vi "Bankomat.vi"() -> ()   [LabVIEW 2021]
uses:
  Stan.ctl
panel:
  in  "Enter":bool
  in  "PIN":string
  in  "Prawe przyciski":T1
  out "Prawe menu":T2
  in  "Lewe przyciski":T1
  out "Lewe menu":T2
  in  "Wprowadź karte":bool
  out "Ekran bankomatu":string
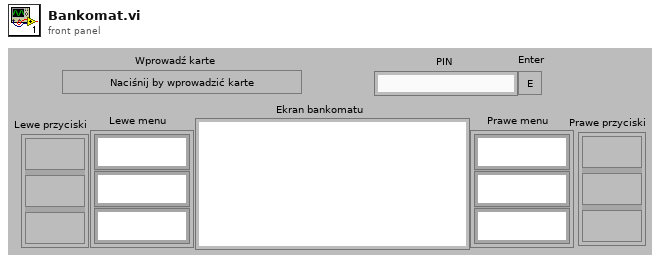
[diagram p1: front panel]
types:
  T1 = cluster{"Func Button":bool, "Func Button 2":bool, "Func Button 3":bool}
  T2 = cluster{"RFS String":string, "RFS String 2":string, "RFS String 3":string}
  T3 = typedef "Stan.ctl" = enum16{"Start", "Idle", "Deposit", "Withdraw", "FastCash", "None", "BalanceInquiry", "ReturnCard"}
  T4 = enum16{"CheckAccountNumber", "ReturnInfo", "Deposit", "Withdraw"}
  T5 = enum8{"Enabled", "Disabled", "Disabled and Grayed Out"}
  T6 = typedef "Konto.ctl" = cluster{"PIN":string, "Imie":string, "Nazwisko":string, "Balans":string}
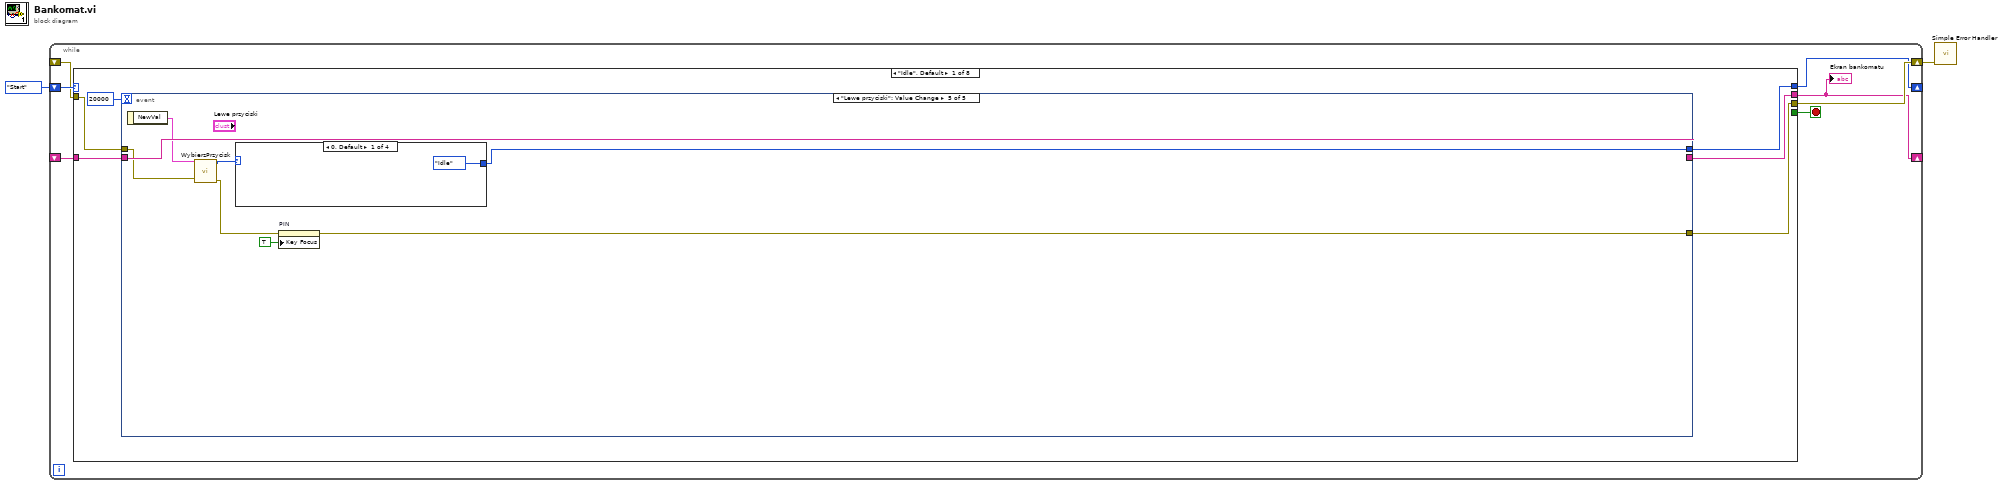
[diagram p0: block diagram]
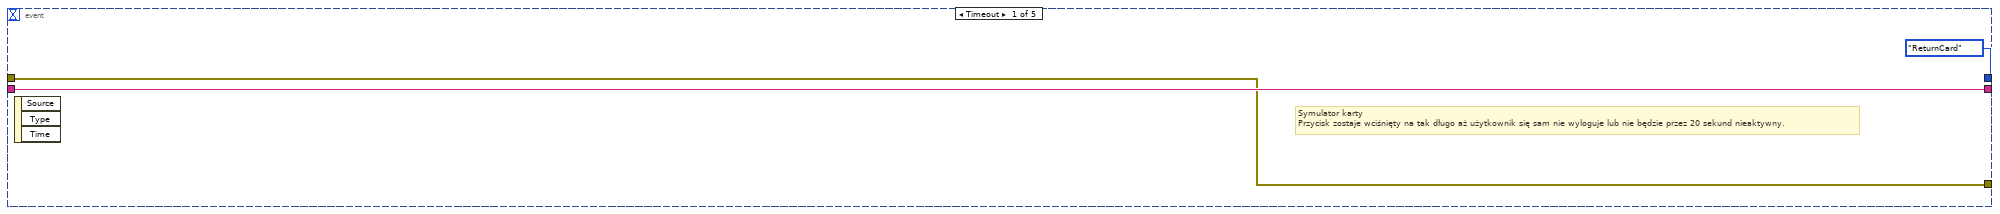
[diagram p2: hidden frame]
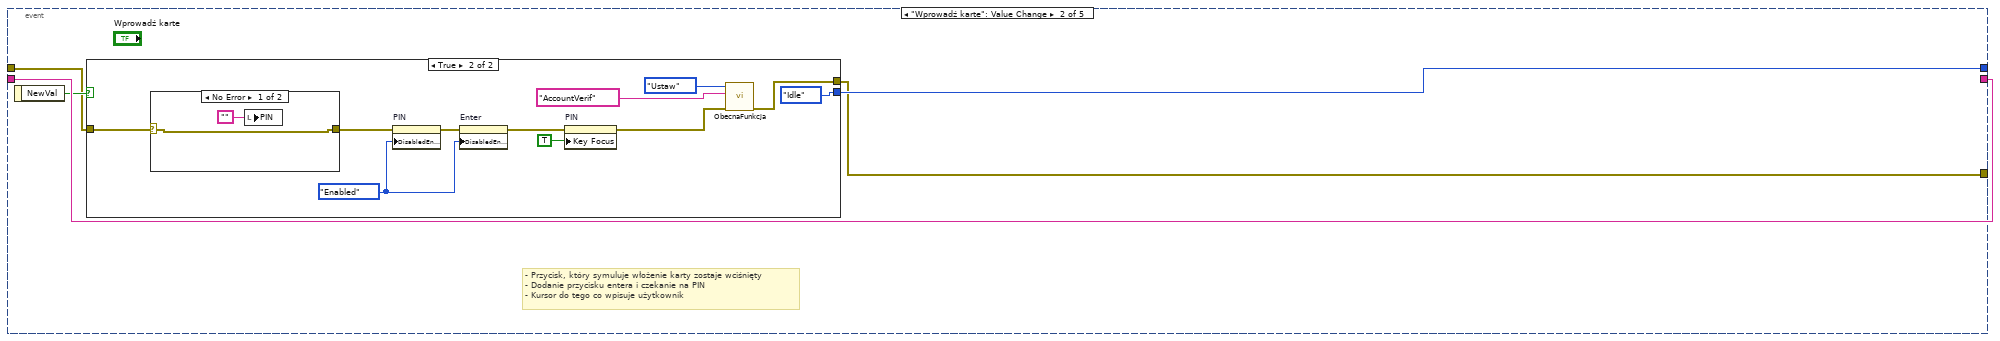
[diagram p3: hidden frame]
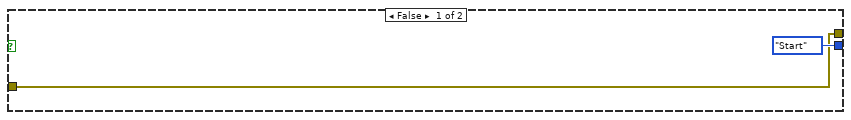
[diagram p4: hidden frame]
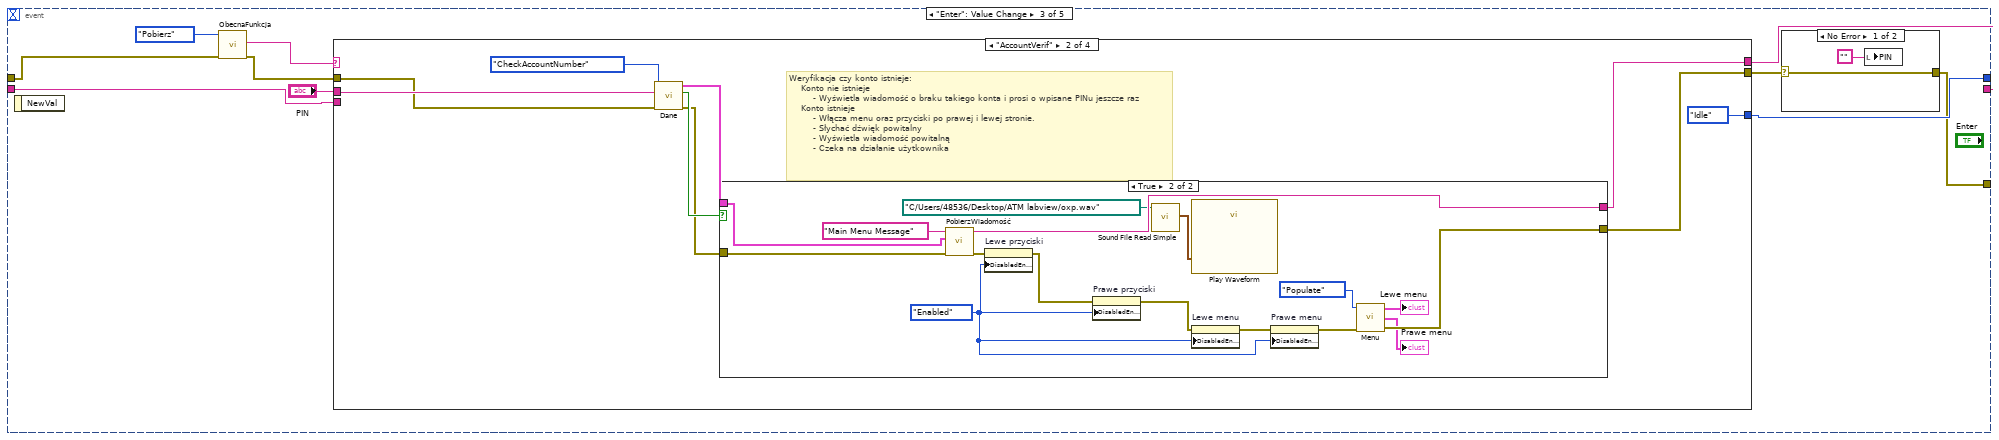
[diagram p6: hidden frame]
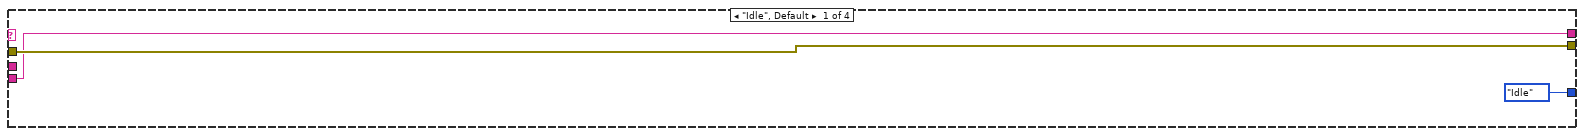
[diagram p8: hidden frame]
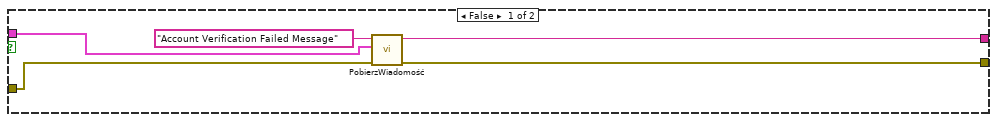
[diagram p9: hidden frame]
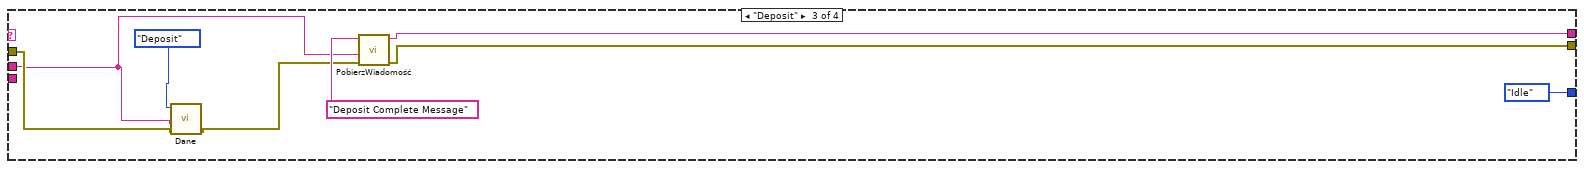
[diagram p10: hidden frame]
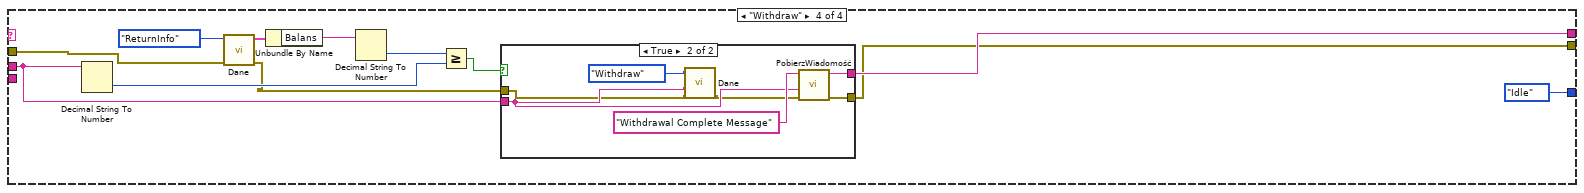
[diagram p11: hidden frame]
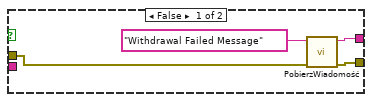
[diagram p12: hidden frame]
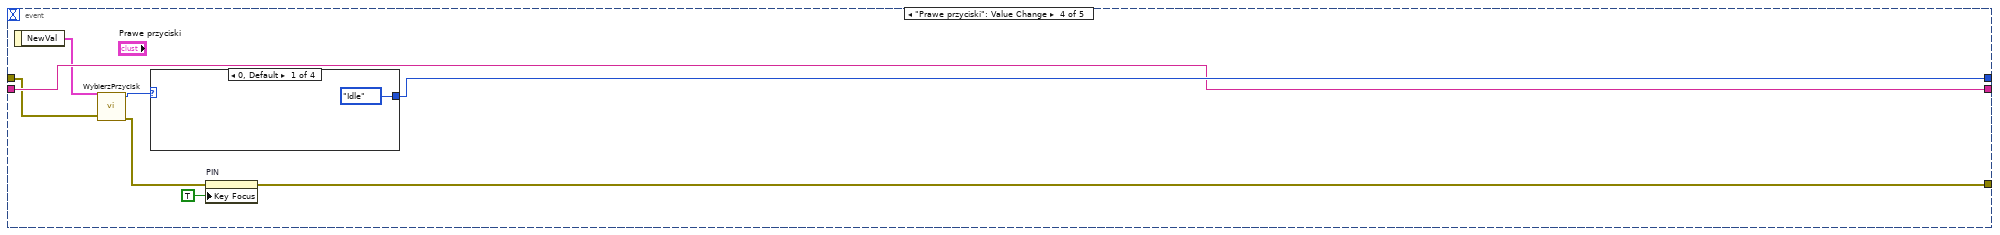
[diagram p13: hidden frame]
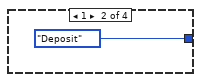
[diagram p14: hidden frame]
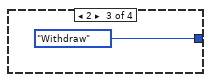
[diagram p15: hidden frame]
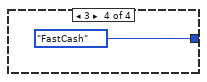
[diagram p16: hidden frame]
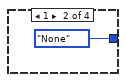
[diagram p17: hidden frame]
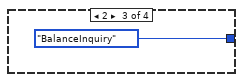
[diagram p18: hidden frame]
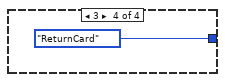
[diagram p19: hidden frame]
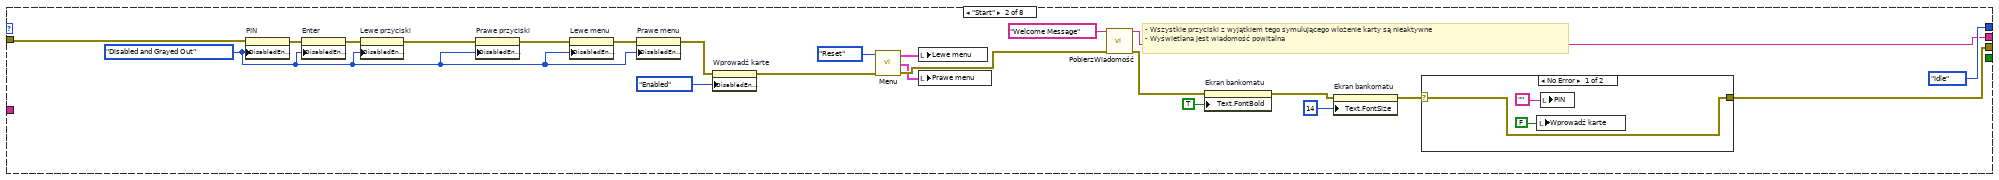
[diagram p20: hidden frame]
diagram:
  n1 = while {
    shift-right: [w3] -> _
    shift-left: Stan."Start" -> [w9]
    shift-right: [w8] -> w1
    shift-left: _ -> [w7]
    shift-right: [w5] -> _
    shift-left: _ -> [w4]
    stop <- w6 stop-if-true
    n2 = case shown="\"Idle\", Default" w9 {
      tunnel: [w12 Stan."Idle" _ Stan."Idle" Stan."Idle" Stan."Idle" Stan."Idle" Stan."Idle"] -> w3
      tunnel: [w13 w142 w180 w203 w212 w222 w241 w248] -> w8
      tunnel: w7 -> [w14 w141 w179 w202 w211 w219 w241 w247]
      tunnel: [_ _ TRUE _ _ _ _ _] -> w6
      tunnel: [w11 w153 w176 w204 w214 w223 "" ("Message") w249] -> w5
      tunnel: w4 -> [w10 _ _ _ _ _ _ _]
      frame "Idle", Default {
        n3 = event shown="[4] \"Lewe przyciski\": Value Change" {
          selector: _ -> [_ _ _ _ _]
          dyn-events: _ -> [_ _ _ _ _]
          timeout: 20000 -> [_ _ _ _ _]
          tunnel: [Stan."ReturnCard" w21 w49 w124 w136] -> w12
          tunnel: w14 -> [w16 w20 w44 w117 w129]
          tunnel: [w16 w19 w41 w121 w133] -> w13
          tunnel: [w17 w23 w46 w123 w135] -> w11
          tunnel: w10 -> [w17 w23 w45 w123 w135]
          event Timeout {
            # "Symulator karty \nPrzycisk zostaje wciśnięty na tak długo aż użytkownik się sam nie wyloguje lub nie będzie przez 20 sekund nieaktywny."
            n4 = event-data() -> ()  [unwired: 1 in, 3 out]
          }
          event "Wprowadź karte": Value Change {
            # "- Przycisk, który symuluje włożenie karty zostaje wciśnięty\n- Dodanie przycisku entera i czekanie na PIN \n- Kursor do tego co wpisuje użytkownik"
            n5 = event-data() -> ("NewVal"=w22:bool)  [unwired: 1 in]
            n6 = case shown="True" w22 {
              tunnel: [Stan."Start" Stan."Idle"] -> w21
              tunnel: w20 -> [w24 w29]
              tunnel: [w24 w27] -> w19
              frame False {
              }
              frame True {
                w36 = T5."Enabled" ("Disabled")
                n7 = case shown="No Error" w29 {
                  selector: w29 -> [w37 w39]
                  tunnel: [w37 w39] -> w28
                  frame No Error {
                    n8 = local write "PIN"("") -> ()
                  }
                  frame Error {
                  }
                }
                n9 = property on="PIN" class="Str"(error in=w28, "DisabledEnum"=w36) -> (error out=w32:errorcluster)  [unwired: 1 in, 1 out]
                n10 = property on="Enter" class="Bool"(error in=w32, "DisabledEnum"=w36) -> (error out=w31:errorcluster)  [unwired: 1 in, 1 out]
                n11 = property on="PIN" class="Str"(error in=w31, "Key Focus"=TRUE) -> (error out=w30:errorcluster)  [unwired: 1 in, 1 out]
                n12 = call "ObecnaFunkcja.vi"("error in"=w30, "Funkcja wejścia"="AccountVerif" ("Function In"), "Akcja"=enum16{"Ustaw", "Pobierz"}."Ustaw") -> ("error out"=w27:errorcluster)  [unwired: 7 in, 1 out]
              }
            }
          }
          event "Enter": Value Change {
            n13 = event-data() -> ()  [unwired: 1 in, 1 out]
            n14 = call "ObecnaFunkcja.vi"("error in"=w44, "Akcja"=enum16{"Ustaw", "Pobierz"}."Pobierz") -> ("error out"=w43:errorcluster, "Funkcja wyjścia"=w48:string)  [unwired: 8 in]
            n15 = case shown="\"AccountVerif\"" w48 {
              tunnel: w43 -> [w54 w60 w89 w94]
              tunnel: [w54 w64 w90 w98] -> w42
              tunnel: [Stan."Idle" Stan."Idle" Stan."Idle" Stan."Idle"] -> w49
              tunnel: "PIN" -> [_ w61 w88 w101]
              tunnel: [w53 w62 w91 w99] -> w46
              tunnel: w45 -> [w53 _ _ _]
              frame "Idle", Default {
              }
              frame "AccountVerif" {
                # "Weryfikacja czy konto istnieje:\n    Konto nie istnieje\n        - Wyświetla wiadomość o braku takiego konta i prosi o wpisane PINu jeszcze raz \n    Konto istnieje \n        - Włącza menu oraz przyciski po prawej i lewej stronie.\n        - Słychać dźwięk powitalny\n        - Wyświetla wiadomość powitalną\n        - Czeka na działanie użytkownika"
                n16 = call "Dane.vi"("error in"=w60, "PIN"=w61, "Enum"=T4."CheckAccountNumber") -> ("error out"=w57:errorcluster, "Konto istniejące"=w58:bool, "Konto"=w59:T6)  [unwired: 6 in]
                n17 = case shown="True" w58 {
                  tunnel: w57 -> [w68 w80]
                  tunnel: [w67 w77] -> w64
                  tunnel: w59 -> [w66 w76]
                  tunnel: [w65 w75] -> w62
                  frame False {
                    n18 = call "PobierzWiadomość.vi"("error in"=w68, "Konto"=w66, "Typ wiadomości"="Account Verification Failed Message" ("Message Type")) -> ("error out"=w67:errorcluster, "Wiadomość"=w65:string)  [unwired: 7 in]
                  }
                  frame True {
                    w81 = T5."Enabled" ("Disabled")
                    n19 = call "PobierzWiadomość.vi"("error in"=w80, "Konto"=w76, "Typ wiadomości"="Main Menu Message" ("Message Type")) -> ("error out"=w79:errorcluster, "Wiadomość"=w75:string)  [unwired: 7 in]
                    n20 = property on="Lewe przyciski" class="Clust"(error in=w79, "DisabledEnum"=w81) -> (error out=w84:errorcluster)  [unwired: 1 in, 1 out]
                    n21 = property on="Prawe przyciski" class="Clust"(error in=w84, "DisabledEnum"=w81) -> (error out=w83:errorcluster)  [unwired: 1 in, 1 out]
                    n22 = call <vilib>:"Sound File Read Simple.vi"("path"=path "C:/Users/48536/Desktop/ATM labview/oxp.wav") -> ("data"=w71:waveform(dbl)[])  [unwired: 7 in, 3 out]
                    n23 = call "Play Waveform"("Data"=w71) -> ()  [unwired: 18 in, 1 out]
                    n24 = property on="Lewe menu" class="Clust (strict)"(error in=w83, "DisabledEnum"=w81) -> (error out=w82:errorcluster)  [unwired: 1 in, 1 out]
                    n25 = property on="Prawe menu" class="Clust (strict)"(error in=w82, "DisabledEnum"=w81) -> (error out=w78:errorcluster)  [unwired: 1 in, 1 out]
                    n26 = call "Menu.vi"("Enum"=enum16{"Reset", "Populate"}."Populate", "error in"=w78) -> ("Lewe menu"=→"Lewe menu":T2, "Prawe menu"=→"Prawe menu":T2, "error out"=w77:errorcluster)  [unwired: 4 in]
                  }
                }
              }
              frame "Deposit" {
                n27 = call "Dane.vi"("error in"=w89, "Ilość"=w88, "Enum"=T4."Deposit") -> ("error out"=w86:errorcluster)  [unwired: 6 in, 2 out]
                n28 = call "PobierzWiadomość.vi"("error in"=w86, "Ilość"=w88, "Typ wiadomości"="Deposit Complete Message") -> ("error out"=w90:errorcluster, "Wiadomość"=w91:string)  [unwired: 7 in]
              }
              frame "Withdraw" {
                n29 = Decimal String To Number(string=w101) -> (number=w103:i32)  [unwired: 2 in, 1 out]
                n30 = call "Dane.vi"("error in"=w94, "Enum"=T4."ReturnInfo") -> ("error out"=w95:errorcluster, "Konto"=w96:T6)  [unwired: 7 in, 1 out]
                n31 = Unbundle By Name(w96) -> ("Balans"=w105:string)
                n32 = Decimal String To Number(string=w105) -> (number=w104:i32)  [unwired: 2 in, 1 out]
                n33 = Greater Or Equal?(x=w104, y=w103) -> (x >= y?=w102:bool)
                n34 = case shown="True" w102 {
                  tunnel: w101 -> [_ w112]
                  tunnel: [w108 w115] -> w99
                  tunnel: w95 -> [w107 w111]
                  tunnel: [w106 w114] -> w98
                  frame False {
                    n35 = call "PobierzWiadomość.vi"("error in"=w107, "Typ wiadomości"="Withdrawal Failed Message" ("ATM Messages")) -> ("error out"=w106:errorcluster, "Wiadomość"=w108:string)  [unwired: 8 in]
                  }
                  frame True {
                    n36 = call "Dane.vi"("error in"=w111, "Ilość"=w112, "Enum"=T4."Withdraw") -> ("error out"=w110:errorcluster)  [unwired: 6 in, 2 out]
                    n37 = call "PobierzWiadomość.vi"("error in"=w110, "Ilość"=w112, "Typ wiadomości"="Withdrawal Complete Message" ("ATM Messages")) -> ("error out"=w114:errorcluster, "Wiadomość"=w115:string)  [unwired: 7 in]
                  }
                }
              }
            }
            n38 = case shown="No Error" w42 {
              selector: w42 -> [w50 w52]
              tunnel: [w50 w52] -> w41
              frame No Error {
                n39 = local write "PIN"("") -> ()
              }
              frame Error {
              }
            }
          }
          event "Prawe przyciski": Value Change {
            n40 = event-data() -> ("NewVal"=w120:T1)  [unwired: 1 in]
            n41 = call "WybierzPrzycisk.vi"("error in"=w117, "Wartość"=w120) -> ("error out"=w118:errorcluster, "Numer"=w119:u32)  [unwired: 8 in]
            n42 = case shown="0, Default" w119 {
              tunnel: [Stan."Idle" Stan."Deposit" Stan."Withdraw" Stan."FastCash"] -> w124
              frame 0, Default {
              }
              frame 1 {
              }
              frame 2 {
              }
              frame 3 {
              }
            }
            n43 = property on="PIN" class="Str"(error in=w118, "Key Focus"=TRUE) -> (error out=w121:errorcluster)  [unwired: 1 in, 1 out]
          }
          event "Lewe przyciski": Value Change {
            n44 = event-data() -> ("NewVal"=w132:T1)  [unwired: 1 in]
            n45 = call "WybierzPrzycisk.vi"("error in"=w129, "Wartość"=w132) -> ("error out"=w130:errorcluster, "Numer"=w131:u32)  [unwired: 8 in]
            n46 = case shown="0, Default" w131 {
              tunnel: [Stan."Idle" Stan."None" Stan."BalanceInquiry" Stan."ReturnCard"] -> w136
              frame 0, Default {
              }
              frame 1 {
              }
              frame 2 {
              }
              frame 3 {
              }
            }
            n47 = property on="PIN" class="Str"(error in=w130, "Key Focus"=TRUE) -> (error out=w133:errorcluster)  [unwired: 1 in, 1 out]
          }
        }
      }
      frame "Start" {
        w162 = T5."Disabled and Grayed Out" ("Disabled")
        # "- Wszystkie przyciski z wyjątkiem tego symulującego wlożenie karty są nieaktywne\n- Wyświetlana jest wiadomość powitalna"
        n48 = property on="PIN" class="Str"(error in=w141, "DisabledEnum"=w162) -> (error out=w159:errorcluster)  [unwired: 1 in, 1 out]
        n49 = property on="Enter" class="Bool"(error in=w159, "DisabledEnum"=w162) -> (error out=w158:errorcluster)  [unwired: 1 in, 1 out]
        n50 = property on="Lewe przyciski" class="Clust"(error in=w158, "DisabledEnum"=w162) -> (error out=w157:errorcluster)  [unwired: 1 in, 1 out]
        n51 = property on="Prawe przyciski" class="Clust"(error in=w157, "DisabledEnum"=w162) -> (error out=w156:errorcluster)  [unwired: 1 in, 1 out]
        n52 = property on="Lewe menu" class="Clust (strict)"(error in=w156, "DisabledEnum"=w162) -> (error out=w155:errorcluster)  [unwired: 1 in, 1 out]
        n53 = property on="Prawe menu" class="Clust (strict)"(error in=w155, "DisabledEnum"=w162) -> (error out=w154:errorcluster)  [unwired: 1 in, 1 out]
        n54 = property on="Wprowadź karte" class="Bool (strict)"(error in=w154, "DisabledEnum"=T5."Enabled" ("Disabled")) -> (error out=w148:errorcluster)  [unwired: 1 in, 1 out]
        n55 = call "Menu.vi"("Enum"=enum16{"Reset", "Populate"}."Reset", "error in"=w148) -> ("Lewe menu"=w150:T2, "Prawe menu"=w149:T2, "error out"=w152:errorcluster)  [unwired: 4 in]
        n56 = local write "Lewe menu"(w150) -> ()
        n57 = local write "Prawe menu"(w149) -> ()
        n58 = call "PobierzWiadomość.vi"("error in"=w152, "Typ wiadomości"="Welcome Message" ("ATM Messages")) -> ("error out"=w147:errorcluster, "Wiadomość"=w153:string)  [unwired: 8 in]
        n59 = property on="Ekran bankomatu" class="Str"(error in=w147, "Text.FontBold"=TRUE ("Text.Font:Bold")) -> (error out=w146:errorcluster)  [unwired: 1 in, 1 out]
        n60 = property on="Ekran bankomatu" class="Str"(error in=w146, "Text.FontSize"=u32 14 ("Text.Font:Size")) -> (error out=w143:errorcluster)  [unwired: 1 in, 1 out]
        n61 = case shown="No Error" w143 {
          selector: w143 -> [w166 w167]
          tunnel: [w166 w167] -> w142
          frame No Error {
            n62 = local write "Wprowadź karte"(FALSE ("Card Simulator")) -> ()
            n63 = local write "PIN"("") -> ()
          }
          frame Error {
          }
        }
      }
      frame "ReturnCard" {
        w192 = T5."Disabled and Grayed Out" ("Disabled")
        # "Po wylogowaniu:\n-Wszystkie przyciski oraz menu przestają być aktywne\n-Przycisk symulujący wkładanie karty staje się znów aktywny\n-Włączany jest dźwięk pożegnalny"
        n64 = property on="PIN" class="Str"(error in=w179, "DisabledEnum"=w192) -> (error out=w190:errorcluster)  [unwired: 1 in, 1 out]
        n65 = property on="Enter" class="Bool"(error in=w190, "DisabledEnum"=w192) -> (error out=w189:errorcluster)  [unwired: 1 in, 1 out]
        n66 = property on="Lewe przyciski" class="Clust"(error in=w189, "DisabledEnum"=w192) -> (error out=w188:errorcluster)  [unwired: 1 in, 1 out]
        n67 = call <vilib>:"Sound File Read Simple.vi"("path"=path "C:/Users/48536/Desktop/ATM labview/end.wav") -> ("data"=w169:waveform(dbl)[])  [unwired: 7 in, 3 out]
        n68 = call "Play Waveform2"("Data"=w169) -> ()  [unwired: 18 in, 1 out]
        n69 = property on="Prawe przyciski" class="Clust"(error in=w188, "DisabledEnum"=w192) -> (error out=w187:errorcluster)  [unwired: 1 in, 1 out]
        n70 = property on="Lewe menu" class="Clust (strict)"(error in=w187, "DisabledEnum"=w192) -> (error out=w186:errorcluster)  [unwired: 1 in, 1 out]
        n71 = property on="Prawe menu" class="Clust (strict)"(error in=w186, "DisabledEnum"=w192) -> (error out=w185:errorcluster)  [unwired: 1 in, 1 out]
        n72 = property on="Wprowadź karte" class="Bool (strict)"(error in=w185, "DisabledEnum"=T5."Enabled" ("Disabled")) -> (error out=w173:errorcluster)  [unwired: 1 in, 1 out]
        n73 = call "Menu.vi"("Enum"=enum16{"Reset", "Populate"}."Reset", "error in"=w173) -> ("Lewe menu"=w172:T2, "Prawe menu"=w171:T2, "error out"=w170:errorcluster)  [unwired: 4 in]
        n74 = local write "Lewe menu"(w172) -> ()
        n75 = local write "Prawe menu"(w171) -> ()
        n76 = call "PobierzWiadomość.vi"("error in"=w170, "Typ wiadomości"="Session Terminate Message" ("ATM Messages")) -> ("error out"=w177:errorcluster, "Wiadomość"=w176:string)  [unwired: 8 in]
        n77 = property on="Ekran bankomatu" class="Str"(error in=w177, "Text.FontBold"=TRUE ("Text.Font:Bold")) -> (error out=w184:errorcluster)  [unwired: 1 in, 1 out]
        n78 = property on="Ekran bankomatu" class="Str"(error in=w184, "Text.FontSize"=u32 14 ("Text.Font:Size")) -> (error out=w181:errorcluster)  [unwired: 1 in, 1 out]
        n79 = case shown="No Error" w181 {
          selector: w181 -> [w195 w196]
          tunnel: [w195 w196] -> w180
          frame No Error {
            n80 = local write "Wprowadź karte"(FALSE ("Card Simulator")) -> ()
            n81 = local write "PIN"("") -> ()
          }
          frame Error {
          }
        }
      }
      frame "Deposit" {
        n82 = case shown="No Error" w202 {
          selector: w202 -> [w208 w209]
          tunnel: [w208 w209] -> w201
          frame No Error {
            n83 = local write "PIN"("") -> ()
            n84 = property on="PIN" class="Str"("Key Focus"=TRUE) -> ()  [unwired: 2 in, 2 out]
          }
          frame Error {
          }
        }
        n85 = call "ObecnaFunkcja.vi"("error in"=w201, "Funkcja wejścia"="Deposit", "Akcja"=enum16{"Ustaw", "Pobierz"}."Ustaw") -> ("error out"=w200:errorcluster)  [unwired: 7 in, 1 out]
        n86 = call "PobierzWiadomość.vi"("error in"=w200, "Typ wiadomości"="Deposit Message") -> ("error out"=w203:errorcluster, "Wiadomość"=w204:string)  [unwired: 8 in]
      }
      frame "Withdraw" {
        n87 = call "ObecnaFunkcja.vi"("error in"=w211, "Funkcja wejścia"="Withdraw" ("Function In"), "Akcja"=enum16{"Ustaw", "Pobierz"}."Ustaw") -> ("error out"=w213:errorcluster)  [unwired: 7 in, 1 out]
        n88 = call "PobierzWiadomość.vi"("error in"=w213, "Typ wiadomości"="Withdrawal Message" ("ATM Messages")) -> ("error out"=w212:errorcluster, "Wiadomość"=w214:string)  [unwired: 8 in]
      }
      frame "FastCash" {
        w224 = "50"
        # "50 zł szybkiej wypłaty"
        n89 = call "Dane.vi"("error in"=w219, "Enum"=T4."ReturnInfo") -> ("error out"=w220:errorcluster, "Konto"=w221:T6)  [unwired: 7 in, 1 out]
        n90 = Unbundle By Name(w221) -> ("Balans"=w228:string)
        n91 = Decimal String To Number(string=w224) -> (number=w225:i32)  [unwired: 2 in, 1 out]
        n92 = Decimal String To Number(string=w228) -> (number=w226:i32)  [unwired: 2 in, 1 out]
        n93 = Greater Or Equal?(x=w226, y=w225) -> (x >= y?=w227:bool)
        n94 = case shown="True" w227 {
          tunnel: [w232 w239] -> w223
          tunnel: w224 -> [_ w235]
          tunnel: w220 -> [w231 w236]
          tunnel: [w230 w238] -> w222
          frame False {
            n95 = call "PobierzWiadomość.vi"("error in"=w231, "Typ wiadomości"="Withdrawal Failed Message" ("ATM Messages")) -> ("error out"=w230:errorcluster, "Wiadomość"=w232:string)  [unwired: 8 in]
          }
          frame True {
            n96 = call "Dane.vi"("error in"=w236, "Ilość"=w235, "Enum"=T4."Withdraw") -> ("error out"=w237:errorcluster)  [unwired: 6 in, 2 out]
            n97 = call "PobierzWiadomość.vi"("error in"=w237, "Ilość"=w235, "Typ wiadomości"="Withdrawal Complete Message" ("ATM Messages")) -> ("error out"=w238:errorcluster, "Wiadomość"=w239:string)  [unwired: 7 in]
          }
        }
      }
      frame "None" {
      }
      frame "BalanceInquiry" {
        n98 = call "Dane.vi"("error in"=w247, "Enum"=T4."ReturnInfo") -> ("error out"=w246:errorcluster, "Konto"=w245:T6)  [unwired: 7 in, 1 out]
        n99 = Unbundle By Name(w245) -> ("Balans"=w250:string)
        n100 = call "PobierzWiadomość.vi"("error in"=w246, "Ilość"=w250, "Typ wiadomości"="Balance Inquiry Message" ("ATM Messages")) -> ("error out"=w248:errorcluster, "Wiadomość"=w249:string)  [unwired: 7 in]
      }
    }
    "Ekran bankomatu" <- w5
  }
  n101 = call <vilib>:"Simple Error Handler.vi"("error in (no error)"=w1) -> ()  [unwired: 4 in, 5 out]
